vi "WriteMessage.vi"   [LabVIEW 2010]
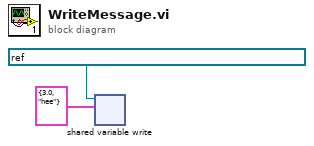
[diagram p0: block diagram]
diagram:
  n1 = shared-variable-write(refnum<k21> "ni.var.psp://My Computer/AcquisitionVariables/Message" ("shared variable refnum in"), cluster{"Channel":dbl, "Message":string} {"Channel"=3.0, "Message"="hee"} ("Message")) -> ()  [unwired: 1 in, 2 out]
